vi "Pololu.Mgr - Set Config Folder.vi"(8 "error in (no error)":errorcluster, 9 "Config Folder":path, 11 "PololuCtrl in":refnum<class "PololuCtrl.lvclass">) -> (0 "error out":errorcluster, 3 "PololuCtrl out":refnum<class "PololuCtrl.lvclass">)   [LabVIEW 2018, in "PololuCtrl.lvclass"]
uses:
  PololuCtrl.lvclass
  PololuCtrl.lvclass/PololuCtrl.ctl
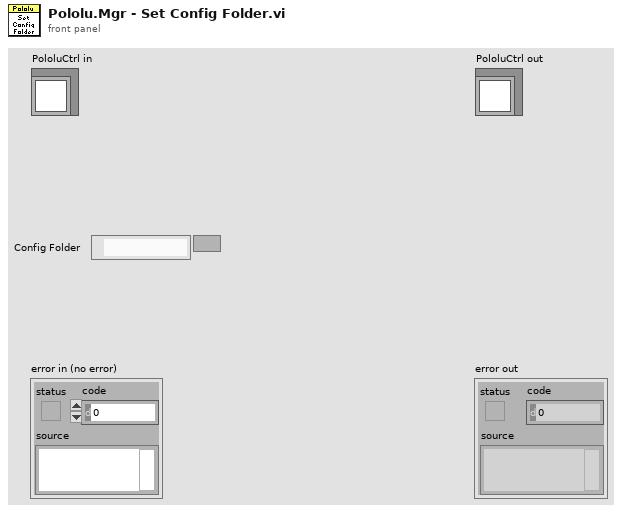
[diagram p1: front panel]
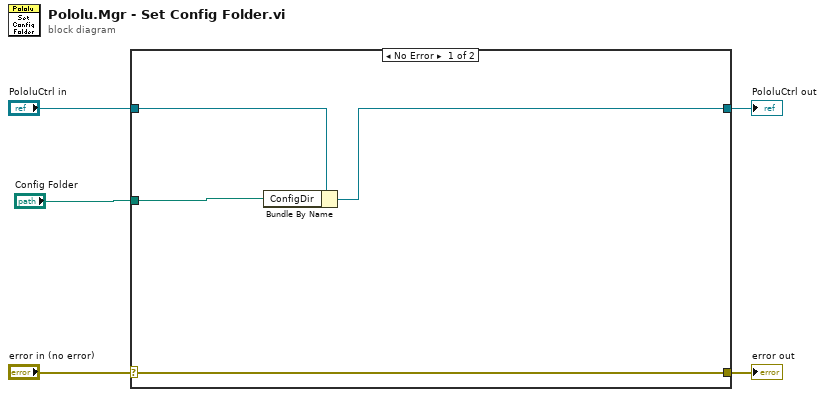
[diagram p0: block diagram]
diagram:
  n1 = case shown="No Error" "error in (no error)" {
    selector: "error in (no error)" -> [w9 w11]
    tunnel: [w9 w11] -> w4
    tunnel: [w7 w10] -> w2
    tunnel: "PololuCtrl in" -> [w6 w10]
    tunnel: "Config Folder" -> [w8 _]
    frame No Error {
      n2 = Bundle By Name(cluster=w6, "ConfigDir"=w8) -> (w7:refnum<class "PololuCtrl.lvclass">)
    }
    frame Error {
    }
  }
  "error out" <- w4
  "PololuCtrl out" <- w2
